vi "Lab Panel V4.85.vi"() -> ()   [LabVIEW 2013]
uses:
  <vilib>/Platform/TimedLoop/XDataNode/timing_clust.ctl
  <vilib>/Platform/TimedLoop/XDataNode/nitl_modes.ctl
  <vilib>/Platform/TimedLoop/XDataNode/wakeup.ctl
  Global display 1.vi
  Global 1.vi
  Global display 3.vi
  Global display 2.vi
  <vilib>/platform/TimedLoop/XDataNode/XDataNode.xnode
  <vilib>/Platform/TimedLoop/XDataNode/XDNodeRunTimeDep.lvlib
panel:
  out "TEMP":bool
  out "AI":bool
  in  "stop all":bool
  in  "ADMIN":bool
  in  "Tab Control 2":T1(tab)
  out "SIG LAB05-2":T2 {"PF" format="%.2f"; "AMPS" format="%.1f"}
  out "SIG LAB05-1":T2 {"PF" format="%.2f"; "AMPS" format="%.1f"}
  out "SIG LAB04-2":T2 {"PF" format="%.2f"; "AMPS" format="%.1f"}
  out "SIG LAB04-1":T2 {"PF" format="%.2f"; "AMPS" format="%.1f"}
  out "SIG LAB03-2":T2 {"PF" format="%.2f"; "AMPS" format="%.1f"}
  out "SIG LAB03-1":T2 {"PF" format="%.2f"; "AMPS" format="%.1f"}
  out "SIG LAB02-2":T2 {"PF" format="%.2f"; "AMPS" format="%.1f"}
  in  "RUN LAB01-1":bool
  in  "O/I  LAB05-1":bool
  in  "O/I  LAB05-2":bool
  in  "O/I  LAB04-1":bool
  in  "O/I  LAB04-2":bool
  in  "O/I  LAB02-1":bool
  in  "O/I  LAB02-2":bool
  in  "O/I  LAB01-2":bool
  in  "O/I  LAB01-1":bool
  in  "O/I  LAB03-1":bool
  in  "RUN LAB05-2":bool
  in  "RUN LAB05-1":bool
  in  "RUN LAB04-2":bool
  in  "RUN LAB04-1":bool
  in  "RUN LAB03-2":bool
  in  "RUN LAB03-1":bool
  in  "RUN LAB02-2":bool
  in  "RUN LAB02-1":bool
  in  "RUN LAB01-2":bool
  in  "SELECT LAB05-2":T3(radio)
  in  "SELECT LAB05-1":T3(radio)
  in  "SELECT LAB04-2":T3(radio)
  in  "SELECT LAB04-1":T3(radio)
  in  "SELECT LAB03-2":T3(radio)
  in  "SELECT LAB03-1":T3(radio)
  in  "SELECT LAB02-2":T3(radio)
  in  "SELECT LAB02-1":T3(radio)
  in  "SELECT LAB01-2":T3(radio)
  in  "SELECT LAB01-1":T3(radio)
  in  "O/I  LAB03-2":bool
  out "SIG LAB01-1":T2 {"PF" format="%.2f"; "AMPS" format="%.1f"}
  out "SIG LAB01-2":T2 {"PF" format="%.2f"; "AMPS" format="%.1f"}
  out "SIG LAB02-1":T2 {"PF" format="%.2f"; "AMPS" format="%.1f"}
  out "DISP LAB05-2":T4 {"MINS" format="%.2g"}
  out "DISP LAB05-1":T4 {"MINS" format="%.2g"}
  out "DISP LAB04-2":T4 {"MINS" format="%.2g"}
  out "DISP LAB04-1":T4 {"MINS" format="%.2g"}
  out "DISP LAB03-2":T4 {"MINS" format="%.2g"}
  out "DISP LAB03-1":T4 {"MINS" format="%.2g"}
  in  "SET LAB05-2":T5={"NAME"="", "DESCRIPTION"="", "CYCLES"=5.0, "T-RISE mins"=0.0, "T-RISE deg C"=0.0} {"CYCLES" min=5.0 step=1.0}
  in  "SET LAB05-1":T5={"NAME"="", "DESCRIPTION"="", "CYCLES"=5.0, "T-RISE mins"=0.0, "T-RISE deg C"=0.0} {"CYCLES" min=5.0 step=1.0}
  in  "SET LAB04-2":T5={"NAME"="", "DESCRIPTION"="", "CYCLES"=5.0, "T-RISE mins"=0.0, "T-RISE deg C"=0.0} {"CYCLES" min=5.0 step=1.0}
  in  "SET LAB04-1":T5={"NAME"="", "DESCRIPTION"="", "CYCLES"=5.0, "T-RISE mins"=0.0, "T-RISE deg C"=0.0} {"CYCLES" min=5.0 step=1.0}
  in  "SET LAB03-2":T5={"NAME"="", "DESCRIPTION"="", "CYCLES"=5.0, "T-RISE mins"=0.0, "T-RISE deg C"=0.0} {"CYCLES" min=5.0 step=1.0}
  in  "SET LAB03-1":T5={"NAME"="", "DESCRIPTION"="", "CYCLES"=5.0, "T-RISE mins"=0.0, "T-RISE deg C"=0.0} {"CYCLES" min=5.0 step=1.0}
  out "DISP LAB02-2":T4 {"MINS" format="%.2g"}
  out "DISP LAB02-1":T4 {"MINS" format="%.2g"}
  in  "SET LAB02-2":T5={"NAME"="", "DESCRIPTION"="", "CYCLES"=5.0, "T-RISE mins"=0.0, "T-RISE deg C"=0.0} {"CYCLES" min=5.0 step=1.0}
  in  "SET LAB02-1":T5={"NAME"="", "DESCRIPTION"="", "CYCLES"=5.0, "T-RISE mins"=0.0, "T-RISE deg C"=0.0} {"CYCLES" min=5.0 step=1.0}
  out "RESULT LAB05-2":bool
  out "RESULT LAB05-1":bool
  out "RESULT LAB04-2":bool
  out "RESULT LAB04-1":bool
  out "RESULT LAB03-2":bool
  out "RESULT LAB03-1":bool
  out "RESULT LAB02-2":bool
  out "RESULT LAB02-1":bool
  out "RESULT LAB01-2":bool
  out "RESULT LAB01-1":bool
  in  "SET LAB01-1":T5={"NAME"="", "DESCRIPTION"="", "CYCLES"=5.0, "T-RISE mins"=0.0, "T-RISE deg C"=0.0} {"CYCLES" min=5.0 step=1.0}
  in  "SET LAB01-2":T5={"NAME"="", "DESCRIPTION"="", "CYCLES"=5.0, "T-RISE mins"=0.0, "T-RISE deg C"=0.0} {"CYCLES" min=5.0 step=1.0}
  out "DISP LAB01-1":T4 {"MINS" format="%.2g"}
  out "DISP LAB01-2":T4 {"MINS" format="%.2f"}
  out "TEMP RISE LAB05-2":cluster{"TL":dbl, "TN":dbl}
  out "TEMP RISE LAB05-1":cluster{"TL":dbl, "TN":dbl}
  out "TEMP RISE LAB04-2":cluster{"TL":dbl, "TN":dbl}
  out "TEMP RISE LAB04-1":cluster{"TL":dbl, "TN":dbl}
  out "TEMP RISE LAB03-2":cluster{"TL":dbl, "TN":dbl}
  out "TEMP RISE LAB03-1":cluster{"TL":dbl, "TN":dbl}
  out "TEMP RISE LAB02-2":cluster{"TL":dbl, "TN":dbl}
  out "TEMP RISE LAB02-1":cluster{"TL":dbl, "TN":dbl}
  out "TEMP RISE LAB01-2":cluster{"TL":dbl, "TN":dbl}
  out "TEMP RISE LAB01-1":cluster{"TL":dbl, "TN":dbl}
  in  "JIG OFF TIME (S)":dbl=2.0 min=2.0 max=10.0 step=0.5 format="%.1g"
  in  "JIG ON TIME (S)":dbl=1.0 min=1.0 max=10.0 step=0.5 format="%.1g"
  out "JIG LAB05-2":bool
  out "JIG LAB05-1":bool
  out "JIG LAB04-2":bool
  out "JIG LAB04-1":bool
  out "JIG LAB03-2":bool
  out "JIG LAB03-1":bool
  out "JIG LAB02-2":bool
  out "JIG LAB02-1":bool
  out "JIG LAB01-2":bool
  out "JIG LAB01-1":bool
  out "TEMP START LAB01-1":cluster{"TL":dbl, "TN":dbl}
  out "TEMP START LAB02-1":cluster{"TL":dbl, "TN":dbl}
  out "TEMP START LAB03-1":cluster{"TL":dbl, "TN":dbl}
  out "TEMP START LAB04-1":cluster{"TL":dbl, "TN":dbl}
  out "TEMP START LAB01-2":cluster{"TL":dbl, "TN":dbl}
  out "TEMP START LAB02-2":cluster{"TL":dbl, "TN":dbl}
  out "TEMP START LAB03-2":cluster{"TL":dbl, "TN":dbl}
  out "TEMP START LAB04-2":cluster{"TL":dbl, "TN":dbl}
  out "TEMP START LAB05-2":cluster{"TL":dbl, "TN":dbl}
  out "TEMP START LAB05-1":cluster{"TL":dbl, "TN":dbl}
  out "LOG LAB05-2":string
  out "LOG LAB04-2":string
  out "LOG LAB03-2":string
  out "LOG LAB02-2":string
  out "LOG LAB01-2":string
  out "LOG LAB05-1":string
  out "LOG LAB04-1":string
  out "LOG LAB03-1":string
  out "LOG LAB02-1":string
  out "LOG LAB01-1":string
  out "TEST VOLTS CHART":dynamicdata(graph)
  in  "Select  Cycle":enum32{"ON CYCLE", "OFF CYCLE"}(radio)
  out "TEST AMPS CHART":dynamicdata(graph)
  out "TEMPERATURE (L) CHART":dynamicdata(graph)
  out "TEMPERATURE (N) CHART":dynamicdata(graph)
  out "Message":string
  in  "MAIL SETTINGS":T6
  out "MAIL REPORT":string
  in  "TO (string):":string
  in  "Send Mail Now":bool
  in  "Auto Mail Send":bool
  in  "Network Directory":path
  out "OFF LO5-1":dbl
  out "OFF LO5-1":dbl
  out "OFF LO4-2":dbl
  out "OFF LO4-1":dbl
  out "OFF LO3-2":dbl
  out "OFF LO3-1":dbl
  out "OFF LO2-1":dbl
  out "OFF LO2-1":dbl
  out "OFF LO1-2":dbl
  out "OFF LO1-1":dbl
  out "JIG RELAY CYCLES":T7
  out "ON L05-2":cluster{"amps":dbl, "volts":dbl, "pf":dbl}
  out "ON L05-1":cluster{"amps":dbl, "volts":dbl, "pf":dbl}
  out "FAIL LAB05-2":cluster{"LO":dbl, "HI":dbl}
  out "FAIL LAB05-1":cluster{"LO":dbl, "HI":dbl}
  out "FAIL LAB04-2":cluster{"LO":dbl, "HI":dbl}
  out "FAIL LAB04-1":cluster{"LO":dbl, "HI":dbl}
  out "FAIL LAB03-2":cluster{"LO":dbl, "HI":dbl}
  out "FAIL LAB03-1":cluster{"LO":dbl, "HI":dbl}
  out "FAIL LAB02-2":cluster{"LO":dbl, "HI":dbl}
  out "FAIL LAB02-1":cluster{"LO":dbl, "HI":dbl}
  out "FAIL LAB01-2":cluster{"LO":dbl, "HI":dbl}
  out "FAIL LAB01-1":cluster{"LO":dbl, "HI":dbl}
  out "ON L01-1":cluster{"amps":dbl, "volts":dbl, "pf":dbl}
  out "ON L01-2":cluster{"amps":dbl, "volts":dbl, "pf":dbl}
  out "ON L02-1":cluster{"amps":dbl, "volts":dbl, "pf":dbl}
  out "ON L02-2":cluster{"amps":dbl, "volts":dbl, "pf":dbl}
  out "ON L03-1":cluster{"amps":dbl, "volts":dbl, "pf":dbl}
  out "ON L03-2":cluster{"amps":dbl, "volts":dbl, "pf":dbl}
  out "ON L04-1":cluster{"amps":dbl, "volts":dbl, "pf":dbl}
  out "ON L04-2":cluster{"amps":dbl, "volts":dbl, "pf":dbl}
  out "TEMP LA05":T8
  out "TEMP LA04":T8
  out "TEMP LA03":T8
  out "TEMP LA02":T8
  out "TEMP LA01":T8
  in  "Test File To":string
  in  "Mail Test Fail":bool
  out "graph flag":bool
  in  "Temp Test Cal":dbl
  in  "spare":dbl
  out "Temp Loops":dbl
  in  "Fail Loops":dbl
  out "Save JC":bool
  out "simulate":bool
  in  "Temp Value":dbl
  in  "Temp Delay Lps":dbl
  in  "SAMPLES":dbl
  in  "RATE (Hz)":dbl
  in  "JIG TEST":T9
  in  "C drive data root dir":path
  out "run lab05-2":bool
  out "run lab05-1":bool
  out "run lab04-2":bool
  out "run lab04-1":bool
  out "run lab03-2":bool
  out "run lab03-1":bool
  out "run lab02-2":bool
  out "run lab02-1":bool
  out "run lab01-2":bool
  out "run lab01-1":bool
  in  "Tab Control":T10(tab)
  out "LAB01-2 (GRAPH)":dynamicdata(graph)
  out "LAB01-1 (GRAPH)":dynamicdata(graph)
  out "LAB02-2 (GRAPH)":dynamicdata(graph)
  out "LAB02-1 (GRAPH)":dynamicdata(graph)
  out "LAB03-2 (GRAPH)":dynamicdata(graph)
  out "LAB03-1 (GRAPH)":dynamicdata(graph)
  out "LAB04-2 (GRAPH)":dynamicdata(graph)
  out "LAB04-1 (GRAPH)":dynamicdata(graph)
  out "LAB05-2 (GRAPH)":dynamicdata(graph)
  out "LAB05-1 (GRAPH)":dynamicdata(graph)
  out "LAB05 TEMP":T11
  out "LAB04 TEMP":T11
  out "LAB02 TEMP":T11
  out "LAB01 TEMP":T11
  out "LAB03 TEMP":T11
  out "Analog Error Array":errorcluster[](array[cluster])
  out "AI loop time":dbl format="%.6g"
  out "loops":dbl
  in  "loop  delay(mS)":dbl
  out "on loops":dbl
  out "off loops":dbl
  out "jig cycle":dbl
  out "TDMS LAB01-1":refnum<k34>
  out "data file error":errorcluster
  out "TDMS LAB02-1":refnum<k34>
  out "TDMS LAB01-2":refnum<k34>
  out "TDMS LAB02-2":refnum<k34>
  out "TDMS LAB03-1":refnum<k34>
  out "TDMS LAB03-2":refnum<k34>
  out "TDMS LAB04-1":refnum<k34>
  out "TDMS LAB04-2":refnum<k34>
  out "TDMS LAB05-1":refnum<k34>
  out "TDMS LAB05-2":refnum<k34>
  out "mail control":string
  out "File Time Stamp":timestamp
  in  "stop":bool
  in  "Select COM port":refnum<visa-resource-name>="COM6"
  out "COM port":refnum<visa-resource-name>="COM6"
  out "CAL LAB01":T12 {"2 (TN) cal" min=0.0 step=0.01 format="%.2f"; "2 (TL) cal" min=0.0 step=0.01 format="%.2f"; "2 (PF) cal" min=0.0 step=0.01 format="%.2f"; "2 (V) cal" min=0.0 step=0.01 format="%.2f"; "2 (A) cal" min=0.0 step=0.01 format="%.2f"; "1 (TN) cal" min=0.0 step=0.01 format="%.2f"; "1 (TL) cal" min=0.0 step=0.01 format="%.2f"; "1 (PF) cal" min=0.0 step=0.01 format="%.2f"; "1 (V) cal" min=0.0 step=0.01 format="%.2f"; "1  (A) cal" min=0.0 step=0.01 format="%.2f"}
  out "CAL LAB03":T12 {"2 (TN) cal" min=0.0 step=0.01 format="%.2f"; "2 (TL) cal" min=0.0 step=0.01 format="%.2f"; "2 (PF) cal" min=0.0 step=0.01 format="%.2f"; "2 (V) cal" min=0.0 step=0.01 format="%.2f"; "2 (A) cal" min=0.0 step=0.01 format="%.2f"; "1 (TN) cal" min=0.0 step=0.01 format="%.2f"; "1 (TL) cal" min=0.0 step=0.01 format="%.2f"; "1 (PF) cal" min=0.0 step=0.01 format="%.2f"; "1 (V) cal" min=0.0 step=0.01 format="%.2f"; "1  (A) cal" min=0.0 step=0.01 format="%.2f"}
  out "CAL LAB02":T13 {"2 (TN) cal" min=0.0 step=0.01 format="%.2f"; "2 (TL) cal" min=0.0 step=0.01 format="%.2f"; "2 (PF) cal" min=0.0 step=0.01 format="%.2f"; "2 (V) cal" min=0.0 step=0.01 format="%.2f"; "2 (A) cal" min=0.0 step=0.01 format="%.2f"; "1 (TN) cal" min=0.0 step=0.01 format="%.2f"; "1 (TL) cal" min=0.0 step=0.01 format="%.2f"; "1 (PF) cal" min=0.0 step=0.01 format="%.2f"; "1 (V) cal" min=0.0 step=0.01 format="%.2f"; "1 (A) cal" min=0.0 step=0.01 format="%.2f"}
  out "CAL LAB05":T12 {"2 (TN) cal" min=0.0 step=0.01 format="%.2f"; "2 (TL) cal" min=0.0 step=0.01 format="%.2f"; "2 (PF) cal" min=0.0 step=0.01 format="%.2f"; "2 (V) cal" min=0.0 step=0.01 format="%.2f"; "2 (A) cal" min=0.0 step=0.01 format="%.2f"; "1 (TN) cal" min=0.0 step=0.01 format="%.2f"; "1 (TL) cal" min=0.0 step=0.01 format="%.2f"; "1 (PF) cal" min=0.0 step=0.01 format="%.2f"; "1 (V) cal" min=0.0 step=0.01 format="%.2f"; "1  (A) cal" min=0.0 step=0.01 format="%.2f"}
  out "CAL LAB04":T12 {"2 (TN) cal" min=0.0 step=0.01 format="%.2f"; "2 (TL) cal" min=0.0 step=0.01 format="%.2f"; "2 (PF) cal" min=0.0 step=0.01 format="%.2f"; "2 (V) cal" min=0.0 step=0.01 format="%.2f"; "2 (A) cal" min=0.0 step=0.01 format="%.2f"; "1 (TN) cal" min=0.0 step=0.01 format="%.2f"; "1 (TL) cal" min=0.0 step=0.01 format="%.2f"; "1 (PF) cal" min=0.0 step=0.01 format="%.2f"; "1 (V) cal" min=0.0 step=0.01 format="%.2f"; "1  (A) cal" min=0.0 step=0.01 format="%.2f"}
  out "cal file error out":errorcluster
  in  "SET (cal)":bool
  # "LAB01"
  # "LAB02"
  # "LAB03"
  # "LAB04"
  # "LAB05"
  # "LAB01"
  # "LAB02"
  # "LAB03"
  # "LAB04"
  # "LAB05"
  # "JIG SET"
  # "PANEL ID / DATE / TIME / DESCRIPTION / CYCLES / TEST TIME / STATUS"
  # "PANEL ID / DATE / TIME / DESCRIPTION / CYCLES / TEST TIME / STATUS"
  # "(Enter recipients address seperated by comma)"
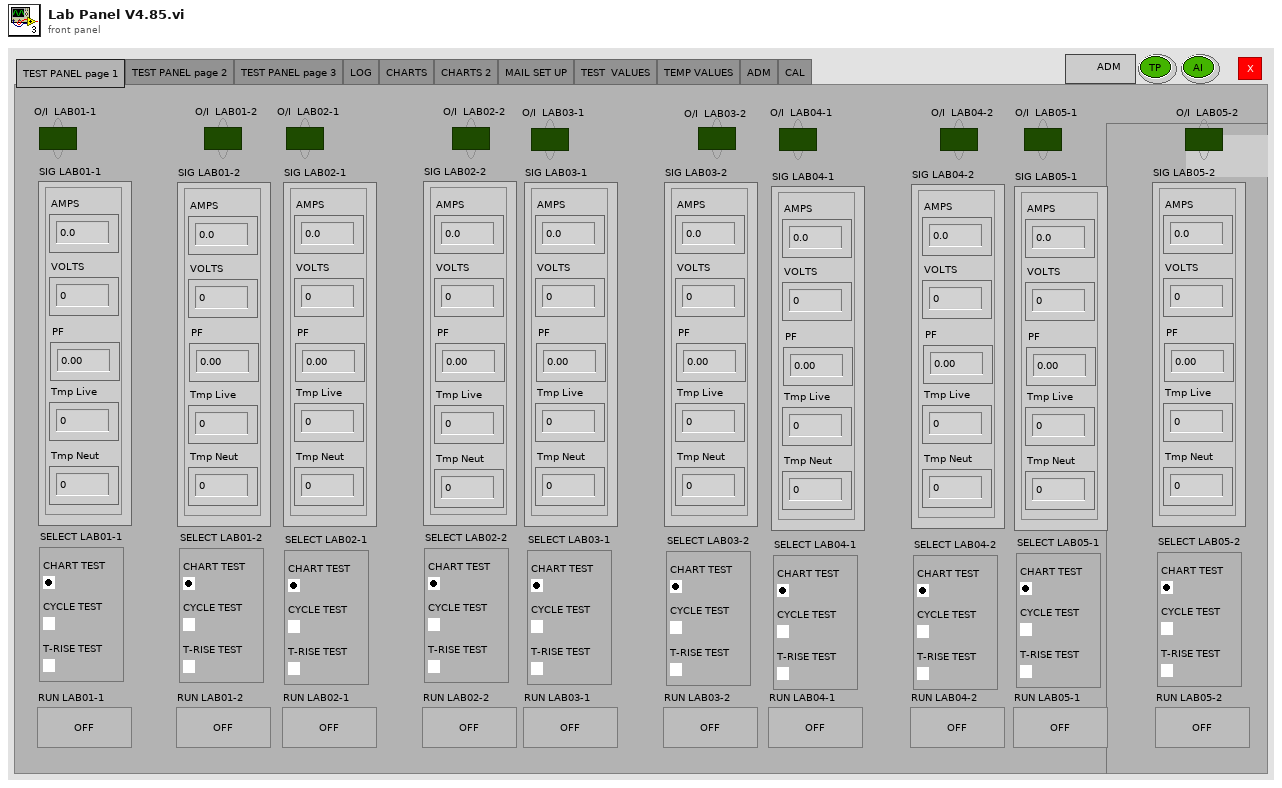
[diagram p1: front panel]
types:
  T1 = enum32{"TEST PANEL page 1", "TEST PANEL page 2", "TEST PANEL page 3", "LOG", "CHARTS", "CHARTS 2", "MAIL SET UP", "TEST  VALUES", "TEMP VALUES", "ADM", "CAL"}
  T2 = cluster{"AMPS":dbl, "VOLTS":dbl, "PF":dbl, "Tmp Live":dbl, "Tmp Neut":dbl}
  T3 = enum32{"CHART TEST", "CYCLE TEST", "T-RISE TEST"}
  T4 = cluster{"CYCLE":dbl, "MINS":dbl, "STATUS":string}
  T5 = cluster{"NAME":string, "DESCRIPTION":string, "CYCLES":dbl, "T-RISE mins":dbl, "T-RISE deg C":dbl}
  T6 = cluster{"OUT SERVER ADDRESS":string, "FROM ACCOUNT":string, "USER NAME":string, "PASSWORD":string, "TEST MAIL":bool, "TEST MAIL STATUS":string, "mail error":errorcluster}
  T7 = cluster{"LAB01-1":dbl, "LAB01-2":dbl, "LAB02-1":dbl, "LAB02-2":dbl, "LAB03-1":dbl, "LAB03-2":dbl, "LAB04-1":dbl, "LAB04-2":dbl, "LAB05-1":dbl, "LAB05-2":dbl}
  T8 = cluster{"TL-1":dbl, "TN-1":dbl, "TL-2":dbl, "TN-2":dbl, "TL -1COUNT":dbl, "TN-1 COUNT":dbl, "TL-2 COUNT":dbl, "TN-2 COUNT":dbl}
  T9 = cluster{" LAB01-1":bool, " LAB01-2":bool, "LAB02-1":bool, " LAB02-2":bool, "LAB03-1":bool, "LAB03-2":bool, "LAB04-1":bool, "LAB04-2":bool, "LAB05-1":bool, "LAB05-2":bool}
  T10 = enum32{"LAB01", "LAB02", "LAB03", "LAB04", "LAB05", "TEMPERATURE", "ERROR"}
  T11 = cluster{"T1 Live":dbl, "T1 Neut":dbl, "T2 Live":dbl, "T2 Neut":dbl, "ID":dbl, "ER":dbl}
  T12 = cluster{"1  (A) cal":dbl, "1 (V) cal":dbl, "1 (PF) cal":dbl, "1 (TL) cal":dbl, "1 (TN) cal":dbl, "2 (A) cal":dbl, "2 (V) cal":dbl, "2 (PF) cal":dbl, "2 (TL) cal":dbl, "2 (TN) cal":dbl}
  T13 = cluster{"1 (A) cal":dbl, "1 (V) cal":dbl, "1 (PF) cal":dbl, "1 (TL) cal":dbl, "1 (TN) cal":dbl, "2 (A) cal":dbl, "2 (V) cal":dbl, "2 (PF) cal":dbl, "2 (TL) cal":dbl, "2 (TN) cal":dbl}
  T14 = enum8{"Enabled", "Disabled", "Disabled and Grayed Out"}
  T15 = typedef "XDNodeRunTimeDep.lvlib/timing_clust.ctl" = cluster{"Expected End [f-1]":u64, "Actual End [f-1]":u64, "Finished Late? [f-1]":bool, "Expected End [i-1]":u64, "Actual End [i-1]":u64, "Finished Late? [i-1]":bool, "Expected Start [i]":u64, "Actual Start [i]":u64, "Expected Start [f]":u64, "Actual Start [f]":u64, "Source Name":string, "Structure Name":string, "Period":i64, "Deadline":i64, "Offset":i64, "Start":i64, "Priority":i32, "Timeout":i32, "Mode":T16, "Wakeup Reason":T17, "Error":errorcluster, "Source Type":string, "Secondary Source Type":string, "Global End Time":u64, "Global Start Time":u64, "Frame Duration":u64, "Iteration Duration":u64, "Assigned CPU":i32, "I/O Scan Engine Mode":u32}
  T16 = typedef "XDNodeRunTimeDep.lvlib/nitl_modes.ctl" = enum32{"No Change", "Process missed periods, maintain original phase", "Discard missed periods, maintain original phase", "Process missed periods, ignore original phase", "Discard missed periods, ignore original phase"}
  T17 = typedef "XDNodeRunTimeDep.lvlib/wakeup.ctl" = enum32{"Normal", "Aborted", "Asynchronous wakeup", "Timing source error", "Timed loop error", "Timeout"}
  T18 = enum16{"open", "open or create", "create or replace", "create", "open (read-only)"}
  T19 = enum16{"open", "replace", "create", "open or create", "replace or create", "replace or create with confirmation"}
  T20 = cluster{"SET LAB01-1":cluster{"NAME":string, "DESCRIPTION":string, "CYCLES":dbl, "T-RISE mins":dbl, "T-RISE deg C":dbl}, "SET LAB01-2":cluster{"NAME":string, "DESCRIPTION":string, "CYCLES":dbl, "T-RISE mins":dbl, "T-RISE deg C":dbl}, "SET LAB02-1":cluster{"NAME":string, "DESCRIPTION":string, "CYCLES":dbl, "T-RISE mins":dbl, "T-RISE deg C":dbl}, "SET LAB02-2":cluster{"NAME":string, "DESCRIPTION":string, "CYCLES":dbl, "T-RISE mins":dbl, "T-RISE deg C":dbl}, "SET LAB03-1":cluster{"NAME":string, "DESCRIPTION":string, "CYCLES":dbl, "T-RISE mins":dbl, "T-RISE deg C":dbl}, "SET LAB03-2":cluster{"NAME":string, "DESCRIPTION":string, "CYCLES":dbl, "T-RISE mins":dbl, "T-RISE deg C":dbl}, "SET LAB04-1":cluster{"NAME":string, "DESCRIPTION":string, "CYCLES":dbl, "T-RISE mins":dbl, "T-RISE deg C":dbl}, "SET LAB04-2":cluster{"NAME":string, "DESCRIPTION":string, "CYCLES":dbl, "T-RISE mins":dbl, "T-RISE deg C":dbl}, "SET LAB05-1":cluster{"NAME":string, "DESCRIPTION":string, "CYCLES":dbl, "T-RISE mins":dbl, "T-RISE deg C":dbl}, "SET LAB05-2":cluster{"NAME":string, "DESCRIPTION":string, "CYCLES":dbl, "T-RISE mins":dbl, "T-RISE deg C":dbl}, "Network Directory":path, "C drive data root dir":path, "RATE (Hz)":dbl, "SAMPLES":dbl, "Select COM port":refnum<visa-resource-name>, "Temp Delay Lps":dbl, "Temp Value":dbl, "Fail Loops":dbl, "Temp Test Cal":dbl, "spare":dbl, "Test File To":string, "Mail Test Fail":bool}
  T21 = cluster{"MAIL SETTINGS":cluster{"OUT SERVER ADDRESS":string, "FROM ACCOUNT":string, "USER NAME":string, "PASSWORD":string, "TEST MAIL":bool, "TEST MAIL STATUS":string, "mail error":errorcluster}, "Auto Mail Send":bool, string}
  T22 = cluster{"T1":dbl, "T2":dbl, "T3":dbl, "T4":dbl, "ID":dbl, "ER":dbl}
  T23 = cluster{"STATUS":string, "OUT SERVER ADDRESS":string, "FROM ACCOUNT":string, "Test File To":string, "Mail Test Fail":bool}
  T24 = cluster{"LAB01-1 (A)":dbl, "LAB01-1 (V)":dbl, "LAB01-1 (PF)":dbl, "LAB01-2 (A)":dbl, "LAB01-2 (V)":dbl, "LAB01-2 (PF)":dbl}
  T25 = cluster{"LAB02-1 (A)":dbl, "LAB02-1 (V)":dbl, "LAB02-1 (PF)":dbl, "LAB02-2 (A)":dbl, "LAB02-2 (V)":dbl, "LAB02-2 (PF)":dbl}
  T26 = cluster{"LAB03-1 (A)":dbl, "LAB03-1 (V)":dbl, "LAB03-1 (PF)":dbl, "LAB03-2 (A)":dbl, "LAB03-2 (V)":dbl, "LAB03-2 (PF)":dbl}
  T27 = cluster{"LAB04-1 (A)":dbl, "LAB04-1 (V)":dbl, "LAB04-1 (PF)":dbl, "LAB04-2 (A)":dbl, "LAB04-2 (V)":dbl, "LAB04-2 (PF)":dbl}
  T28 = cluster{"LAB05-1 (A)":dbl, "LAB05-1 (V)":dbl, "LAB05-1 (PF)":dbl, "LAB05-2 (A)":dbl, "LAB05-2 (V)":dbl, "LAB05-2 (PF)":dbl}
  T29 = cluster{"FAIL LAB01-1":cluster{"LO":dbl, "HI":dbl}, "SIG LAB01-1":cluster{"AMPS":dbl, "VOLTS":dbl, "PF":dbl, "Tmp Live":dbl, "Tmp Neut":dbl}, "TEMP START LAB01-1":cluster{"TL":dbl, "TN":dbl}, "DISP LAB01-1":cluster{"CYCLE":dbl, "MINS":dbl, "STATUS":string}, "SET LAB01-1":cluster{"NAME":string, "DESCRIPTION":string, "CYCLES":dbl, "T-RISE mins":dbl, "T-RISE deg C":dbl}, "TDMS LAB01-1":refnum<k34>}
  T30 = cluster{"FAIL LAB01-2":cluster{"LO":dbl, "HI":dbl}, "SIG LAB01-2":cluster{"AMPS":dbl, "VOLTS":dbl, "PF":dbl, "Tmp Live":dbl, "Tmp Neut":dbl}, "TEMP START LAB01-2":cluster{"TL":dbl, "TN":dbl}, "DISP LAB01-2":cluster{"CYCLE":dbl, "MINS":dbl, "STATUS":string}, "SET LAB01-2":cluster{"NAME":string, "DESCRIPTION":string, "CYCLES":dbl, "T-RISE mins":dbl, "T-RISE deg C":dbl}, "TDMS LAB01-2":refnum<k34>}
  T31 = cluster{"FAIL LAB02-1":cluster{"LO":dbl, "HI":dbl}, "SIG LAB02-1":cluster{"AMPS":dbl, "VOLTS":dbl, "PF":dbl, "Tmp Live":dbl, "Tmp Neut":dbl}, "TEMP START LAB02-1":cluster{"TL":dbl, "TN":dbl}, "DISP LAB02-1":cluster{"CYCLE":dbl, "MINS":dbl, "STATUS":string}, "SET LAB02-1":cluster{"NAME":string, "DESCRIPTION":string, "CYCLES":dbl, "T-RISE mins":dbl, "T-RISE deg C":dbl}, "TDMS LAB02-1":refnum<k34>}
  T32 = cluster{"FAIL LAB02-2":cluster{"LO":dbl, "HI":dbl}, "SIG LAB02-2":cluster{"AMPS":dbl, "VOLTS":dbl, "PF":dbl, "Tmp Live":dbl, "Tmp Neut":dbl}, "TEMP START LAB02-2":cluster{"TL":dbl, "TN":dbl}, "DISP LAB02-2":cluster{"CYCLE":dbl, "MINS":dbl, "STATUS":string}, "SET LAB02-2":cluster{"NAME":string, "DESCRIPTION":string, "CYCLES":dbl, "T-RISE mins":dbl, "T-RISE deg C":dbl}, "TDMS LAB02-2":refnum<k34>}
  T33 = cluster{"FAIL LAB03-1":cluster{"LO":dbl, "HI":dbl}, "SIG LAB03-1":cluster{"AMPS":dbl, "VOLTS":dbl, "PF":dbl, "Tmp Live":dbl, "Tmp Neut":dbl}, "TEMP START LAB03-1":cluster{"TL":dbl, "TN":dbl}, "DISP LAB03-1":cluster{"CYCLE":dbl, "MINS":dbl, "STATUS":string}, "SET LAB03-1":cluster{"NAME":string, "DESCRIPTION":string, "CYCLES":dbl, "T-RISE mins":dbl, "T-RISE deg C":dbl}, "TDMS LAB03-1":refnum<k34>}
  T34 = cluster{"FAIL LAB03-2":cluster{"LO":dbl, "HI":dbl}, "SIG LAB03-2":cluster{"AMPS":dbl, "VOLTS":dbl, "PF":dbl, "Tmp Live":dbl, "Tmp Neut":dbl}, "TEMP START LAB03-2":cluster{"TL":dbl, "TN":dbl}, "DISP LAB03-2":cluster{"CYCLE":dbl, "MINS":dbl, "STATUS":string}, "SET LAB03-2":cluster{"NAME":string, "DESCRIPTION":string, "CYCLES":dbl, "T-RISE mins":dbl, "T-RISE deg C":dbl}, "TDMS LAB03-2":refnum<k34>}
  T35 = cluster{"FAIL LAB04-1":cluster{"LO":dbl, "HI":dbl}, "SIG LAB04-1":cluster{"AMPS":dbl, "VOLTS":dbl, "PF":dbl, "Tmp Live":dbl, "Tmp Neut":dbl}, "TEMP START LAB04-1":cluster{"TL":dbl, "TN":dbl}, "DISP LAB04-1":cluster{"CYCLE":dbl, "MINS":dbl, "STATUS":string}, "SET LAB04-1":cluster{"NAME":string, "DESCRIPTION":string, "CYCLES":dbl, "T-RISE mins":dbl, "T-RISE deg C":dbl}, "TDMS LAB04-1":refnum<k34>}
  T36 = cluster{"FAIL LAB04-2":cluster{"LO":dbl, "HI":dbl}, "SIG LAB04-2":cluster{"AMPS":dbl, "VOLTS":dbl, "PF":dbl, "Tmp Live":dbl, "Tmp Neut":dbl}, "TEMP START LAB04-2":cluster{"TL":dbl, "TN":dbl}, "DISP LAB04-2":cluster{"CYCLE":dbl, "MINS":dbl, "STATUS":string}, "SET LAB04-2":cluster{"NAME":string, "DESCRIPTION":string, "CYCLES":dbl, "T-RISE mins":dbl, "T-RISE deg C":dbl}, "TDMS LAB04-2":refnum<k34>}
  T37 = cluster{"FAIL LAB05-1":cluster{"LO":dbl, "HI":dbl}, "SIG LAB05-1":cluster{"AMPS":dbl, "VOLTS":dbl, "PF":dbl, "Tmp Live":dbl, "Tmp Neut":dbl}, "TEMP START LAB05-1":cluster{"TL":dbl, "TN":dbl}, "DISP LAB05-1":cluster{"CYCLE":dbl, "MINS":dbl, "STATUS":string}, "SET LAB05-1":cluster{"NAME":string, "DESCRIPTION":string, "CYCLES":dbl, "T-RISE mins":dbl, "T-RISE deg C":dbl}, "TDMS LAB05-1":refnum<k34>}
  T38 = cluster{"FAIL LAB05-2":cluster{"LO":dbl, "HI":dbl}, "SIG LAB05-2":cluster{"AMPS":dbl, "VOLTS":dbl, "PF":dbl, "Tmp Live":dbl, "Tmp Neut":dbl}, "TEMP START LAB05-2":cluster{"TL":dbl, "TN":dbl}, "DISP LAB05-2":cluster{"CYCLE":dbl, "MINS":dbl, "STATUS":string}, "SET LAB05-2":cluster{"NAME":string, "DESCRIPTION":string, "CYCLES":dbl, "T-RISE mins":dbl, "T-RISE deg C":dbl}, "TDMS LAB05-2":refnum<k34>}
  T39 = cluster{"MAIL SETTINGS":cluster{"OUT SERVER ADDRESS":string, "FROM ACCOUNT":string, "USER NAME":string, "PASSWORD":string, "TEST MAIL":bool, "TEST MAIL STATUS":string, "mail error":errorcluster}, "Auto Mail Send":bool, "TO (string):":string}
  T40 = cluster{"TP1-L":dbl, "TP1-N":dbl, "TP2-L":dbl, "TP2-N":dbl, "TP1-L COUNT":dbl, "TP1-N COUNT":dbl, "TP2-L COUNT":dbl, "TP2-N COUNT":dbl}
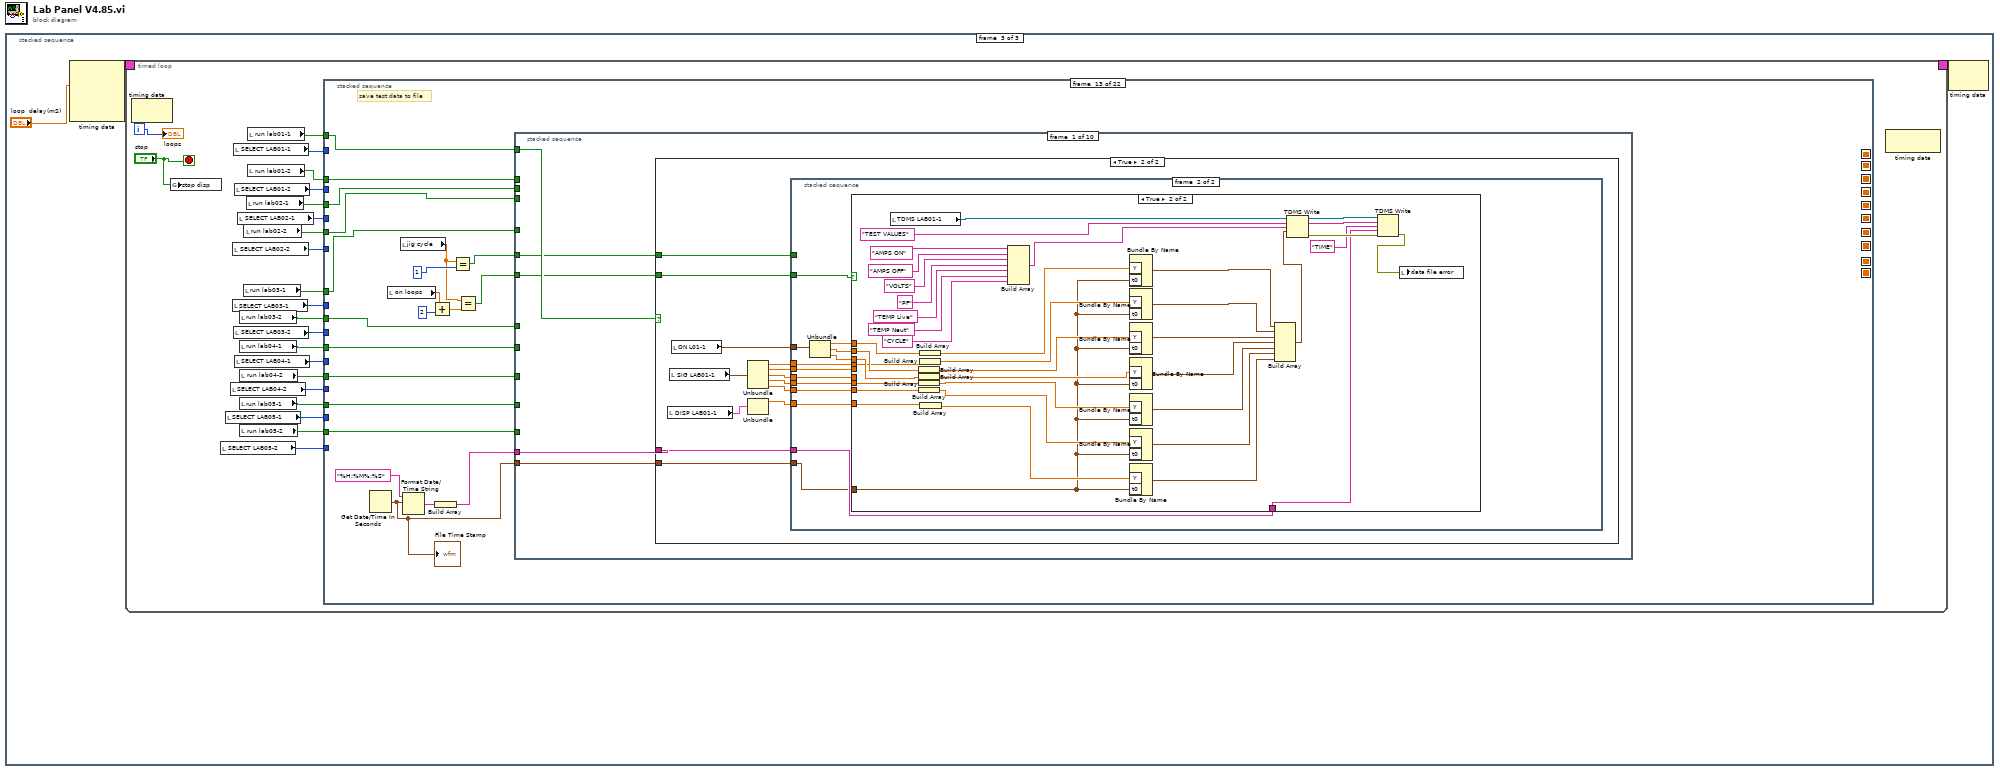
[diagram p0: block diagram]
diagram:
  n1 = stacked-sequence {
    frame #0 {
      n2 = local write "loop  delay(mS)"(500) -> ()
      n3 = local write "Save JC"(FALSE) -> ()
      "jig cycle" <- 0
    }
    frame #1 {
      # "do 1st time set up"
      n4 = stacked-sequence {
        frame #0 {
          # "disable front panel while 1st time set up is being done"
          n5 = disable-structure shown="Enabled" {
            frame Enabled {
              n6 = property on="Tab Control 2" class="TabCtl (strict)"() -> ("Pages"=w10:refnum<vi>[])  [unwired: 2 in, 2 out]
              n7 = Index Array(array=w10, index=9) -> (element=w8:refnum<vi>)
              n8 = property class="Page"(reference=w8, "PageVis"=FALSE) -> ()  [unwired: 1 in, 2 out]
            }
            frame Disabled {
            }
          }
          n9 = property on="Tab Control 2" class="TabCtl (strict)"("Value"=0) -> ()  [unwired: 2 in, 2 out]
          n10 = local write "ADMIN"(FALSE) -> ()
          n11 = property on="Tab Control 2" class="TabCtl (strict)"("DisabledEnum"=T14."Disabled and Grayed Out" ("Disabled")) -> ()  [unwired: 2 in, 2 out]
        }
        frame #1 {
          # "get calibration values"
          n12 = call "sub vi - get calibration values v1.vi"() -> ("LAB01 (CAL)"=→"CAL LAB01":T12, "LAB02 (CAL)"=→"CAL LAB02":T13, "LAB03 (CAL)"=→"CAL LAB03":T12, "LAB04 (CAL)"=→"CAL LAB04":T12, "calibration file error out"=→"cal file error out":errorcluster, "LAB05 (CAL)"=→"CAL LAB05":T12)  [unwired: 10 in]
        }
        frame #2 {
          # "get last saved test settings from file"
          n13 = local read "Network Directory"() -> (w39:path)
          n14 = local read "C drive data root dir"() -> (w37:path)
          n15 = local read "SET LAB05-2"() -> (w69:T5)
          n16 = local read "SET LAB05-1"() -> (w70:T5)
          n17 = local read "SAMPLES"() -> (w35:dbl)
          n18 = local read "SET LAB04-2"() -> (w71:T5)
          n19 = local read "RATE (Hz)"() -> (w36:dbl)
          n20 = local read "SET LAB03-2"() -> (w68:T5)
          n21 = local read "SET LAB04-1"() -> (w72:T5)
          n22 = local read "SET LAB03-1"() -> (w67:T5)
          n23 = local read "SET LAB02-2"() -> (w66:T5)
          n24 = local read "SET LAB02-1"() -> (w65:T5)
          n25 = local read "SET LAB01-2"() -> (w64:T5)
          n26 = local read "SET LAB01-1"() -> (w63:T5)
          n27 = local read "Select COM port"() -> (w31:refnum<visa-resource-name>)
          n28 = local read "Temp Delay Lps"() -> (w30:dbl)
          n29 = local read "Temp Value"() -> (w29:dbl)
          n30 = local read "Temp Test Cal"() -> (w24:dbl)
          n31 = local read "Test File To"() -> (w20:string)
          n32 = local read "Fail Loops"() -> (w26:dbl)
          n33 = local read "Mail Test Fail"() -> (w18:bool)
          n34 = local read "spare"() -> (w23:dbl)
          n35 = Bundle("SET LAB01-1"=w63, "SET LAB01-2"=w64, "SET LAB02-1"=w65, "SET LAB02-2"=w66, "SET LAB03-1"=w67, "SET LAB03-2"=w68, "SET LAB04-1"=w72, "SET LAB04-2"=w71, "SET LAB05-1"=w70, "SET LAB05-2"=w69, "Network Directory"=w39, "C drive data root dir"=w37, "RATE (Hz)"=w36, "SAMPLES"=w35, "Select COM port"=w31, "Temp Delay Lps"=w30, "Temp Value"=w29, "Fail Loops"=w26, "Temp Test Cal"=w24, "spare"=w23, "Test File To"=w20, "Mail Test Fail"=w18) -> (w56:T20)  [unwired: 1 in]
          n36 = String To Path(string="c:\\crabtree\\Set Up\\") -> (path=w60:path)
          n37 = Build Path(base path=w60, name or relative path="settings.bin") -> (appended path=w58:path)
          n38 = Create Folder(path (use dialog)=w60) -> (error out=w62:errorcluster)  [unwired: 2 in, 2 out]
          n39 = call <vilib>:"Clear Errors.vi"("error in (no error)"=w62) -> ()  [unwired: 6 in, 1 out]
          n40 = Open/Create/Replace File(file path (use dialog)=w58) -> (refnum out=w55:refnum<file>, error out=w57:errorcluster)  [unwired: 5 in, 1 out]
          n41 = Read from Binary File(5:w56, 8:w57, 11:w55) -> (0:w52:errorcluster, 2:w54:T20, 3:w53:refnum<file>)  [unwired: 3 in, 1 out]
          n42 = Unbundle(w54) -> ("SET LAB01-1"=w50:T5, "SET LAB01-2"=w49:T5, "SET LAB02-1"=w48:T5, "SET LAB02-2"=w47:T5, "SET LAB03-1"=w46:T5, "SET LAB03-2"=w45:T5, "SET LAB04-1"=w44:T5, "SET LAB04-2"=w43:T5, "SET LAB05-1"=w42:T5, "SET LAB05-2"=w41:T5, "Network Directory"=w40:path, "C drive data root dir"=w38:path, "RATE (Hz)"=w33:dbl, "SAMPLES"=w34:dbl, "Select COM port"=w32:refnum<visa-resource-name>, "Temp Delay Lps"=w28:dbl, "Temp Value"=w27:dbl, "Fail Loops"=w25:dbl, "Temp Test Cal"=w22:dbl, "spare"=w21:dbl, "Test File To"=w19:string, "Mail Test Fail"=w17:bool)
          n43 = Close File(refnum=w53, error in=w52) -> (error out=w51:errorcluster)  [unwired: 1 out]
          n44 = local write "data file error"(w51) -> ()
          n45 = local write "Temp Test Cal"(w22) -> ()
          n46 = local write "Mail Test Fail"(w17) -> ()
          n47 = local write "Test File To"(w19) -> ()
          n48 = local write "Fail Loops"(w25) -> ()
          n49 = local write "Temp Delay Lps"(w28) -> ()
          n50 = local write "C drive data root dir"(w38) -> ()
          n51 = local write "spare"(w21) -> ()
          n52 = local write "Temp Value"(w27) -> ()
          n53 = local write "Select COM port"(w32) -> ()
          n54 = local write "Network Directory"(w40) -> ()
          n55 = local write "SAMPLES"(w34) -> ()
          n56 = local write "RATE (Hz)"(w33) -> ()
          n57 = local write "SET LAB04-2"(w43) -> ()
          n58 = local write "SET LAB05-1"(w42) -> ()
          n59 = local write "SET LAB04-1"(w44) -> ()
          n60 = local write "SET LAB05-2"(w41) -> ()
          n61 = local write "SET LAB02-1"(w48) -> ()
          n62 = local write "SET LAB02-2"(w47) -> ()
          n63 = local write "SET LAB03-1"(w46) -> ()
          n64 = local write "SET LAB03-2"(w45) -> ()
          n65 = local write "SET LAB01-1"(w50) -> ()
          n66 = local write "SET LAB01-2"(w49) -> ()
        }
        frame #3 {
          # "get last saved jig cycles value from file"
          n67 = String To Path(string="c:\\crabtree\\Jig Cycles\\") -> (path=w82:path)
          n68 = Build Path(base path=w82, name or relative path="jigcycles.bin") -> (appended path=w80:path)
          n69 = Create Folder(path (use dialog)=w82) -> (error out=w84:errorcluster)  [unwired: 2 in, 2 out]
          n70 = call <vilib>:"Clear Errors.vi"("error in (no error)"=w84) -> ()  [unwired: 6 in, 1 out]
          n71 = Open/Create/Replace File(file path (use dialog)=w80) -> (refnum out=w78:refnum<file>, error out=w79:errorcluster)  [unwired: 5 in, 1 out]
          n72 = Read from Binary File(5:T7 {"LAB01-1"=0.0, "LAB01-2"=0.0, "LAB02-1"=0.0, "LAB02-2"=0.0, "LAB03-1"=0.0, "LAB03-2"=0.0, "LAB04-1"=0.0, "LAB04-2"=0.0, "LAB05-1"=0.0, "LAB05-2"=0.0} ("JIG RELAY CYCLES"), 8:w79, 11:w78) -> (0:w76:errorcluster, 2:w73:T7, 3:w77:refnum<file>)  [unwired: 3 in, 1 out]
          n73 = local write "JIG RELAY CYCLES"(w73) -> ()
          n74 = Close File(refnum=w77, error in=w76) -> (error out=w75:errorcluster)  [unwired: 1 out]
          n75 = local write "data file error"(w75) -> ()
        }
        frame #4 {
          # "get mail settings"
          n76 = local read "Auto Mail Send"() -> (w88:bool)
          n77 = local read "MAIL SETTINGS"() -> (w92:T6)
          n78 = String To Path(string="c:\\crabtree\\Set Up\\") -> (path=w100:path)
          n79 = Build Path(base path=w100, name or relative path="mail.bin") -> (appended path=w98:path)
          n80 = Create Folder(path (use dialog)=w100) -> (error out=w102:errorcluster)  [unwired: 2 in, 2 out]
          n81 = Bundle("MAIL SETTINGS"=w92, "Auto Mail Send"=w88, "") -> (w91:T21)  [unwired: 1 in]
          n82 = call <vilib>:"Clear Errors.vi"("error in (no error)"=w102) -> ()  [unwired: 6 in, 1 out]
          n83 = Open/Create/Replace File(file path (use dialog)=w98) -> (refnum out=w96:refnum<file>, error out=w97:errorcluster)  [unwired: 5 in, 1 out]
          n84 = Read from Binary File(5:w91, 8:w97, 11:w96) -> (0:w94:errorcluster, 2:w90:T21, 3:w95:refnum<file>)  [unwired: 3 in, 1 out]
          n85 = Unbundle(w90) -> ("MAIL SETTINGS"=w89:T6, "Auto Mail Send"=w87:bool, w86:string)
          n86 = local write "TO (string):"(w86) -> ()
          n87 = local write "Auto Mail Send"(w87) -> ()
          n88 = local write "MAIL SETTINGS"(w89) -> ()
          n89 = Close File(refnum=w95, error in=w94) -> (error out=w93:errorcluster)  [unwired: 1 out]
          n90 = local write "data file error"(w93) -> ()
        }
        frame #5 {
          # "set display status if blank"
          n91 = local read "DISP LAB03-2"() -> (w132:T4)
          n92 = local read "DISP LAB03-1"() -> (w139:T4)
          n93 = local read "DISP LAB02-2"() -> (w146:T4)
          n94 = local read "DISP LAB01-2"() -> (w159:T4)
          n95 = local read "DISP LAB01-1"() -> (w168:T4)
          n96 = local read "DISP LAB02-1"() -> (w153:T4)
          n97 = Unbundle(w132) -> ("STATUS"=w134:string)  [unwired: 2 out]
          n98 = Unbundle(w139) -> ("STATUS"=w141:string)  [unwired: 2 out]
          n99 = Unbundle(w146) -> ("STATUS"=w148:string)  [unwired: 2 out]
          n100 = Unbundle(w153) -> ("STATUS"=w155:string)  [unwired: 2 out]
          n101 = Unbundle(w159) -> ("STATUS"=w162:string)  [unwired: 2 out]
          n102 = Unbundle(w168) -> ("STATUS"=w169:string)  [unwired: 2 out]
          n103 = Equal?(x="", y=w134) -> (x = y?=w136:bool)
          n104 = Equal?(x="", y=w141) -> (x = y?=w143:bool)
          n105 = Equal?(x="", y=w148) -> (x = y?=w150:bool)
          n106 = Equal?(x="", y=w155) -> (x = y?=w157:bool)
          n107 = Equal?(x="", y=w162) -> (x = y?=w164:bool)
          n108 = Equal?(x="", y=w169) -> (x = y?=w171:bool)
          n109 = Select(t="STOP", s=w136, f=w134) -> (s? t:f=w133:string)
          n110 = Select(t="STOP", s=w143, f=w141) -> (s? t:f=w140:string)
          n111 = Select(t="STOP", s=w150, f=w148) -> (s? t:f=w147:string)
          n112 = Select(t="STOP", s=w157, f=w155) -> (s? t:f=w154:string)
          n113 = Select(t="STOP", s=w164, f=w162) -> (s? t:f=w161:string)
          n114 = Select(t="STOP", s=w171, f=w169) -> (s? t:f=w167:string)
          n115 = Bundle(cluster=w132, "STATUS"=w133) -> (w131:T4)  [unwired: 2 in]
          n116 = Bundle(cluster=w139, "STATUS"=w140) -> (w138:T4)  [unwired: 2 in]
          n117 = Bundle(cluster=w146, "STATUS"=w147) -> (w145:T4)  [unwired: 2 in]
          n118 = Bundle(cluster=w153, "STATUS"=w154) -> (w152:T4)  [unwired: 2 in]
          n119 = Bundle(cluster=w159, "STATUS"=w161) -> (w160:T4)  [unwired: 2 in]
          n120 = Bundle(cluster=w168, "STATUS"=w167) -> (w166:T4)  [unwired: 2 in]
          n121 = local write "DISP LAB01-2"(w160) -> ()
          n122 = local write "DISP LAB01-1"(w166) -> ()
          n123 = local write "DISP LAB02-1"(w152) -> ()
          n124 = local write "DISP LAB03-1"(w138) -> ()
          n125 = local write "DISP LAB02-2"(w145) -> ()
          n126 = local write "DISP LAB03-2"(w131) -> ()
          n127 = local read "DISP LAB05-2"() -> (w104:T4)
          n128 = local read "DISP LAB05-1"() -> (w111:T4)
          n129 = local read "DISP LAB04-2"() -> (w113:T4)
          n130 = local read "DISP LAB04-1"() -> (w115:T4)
          n131 = Unbundle(w104) -> ("STATUS"=w106:string)  [unwired: 2 out]
          n132 = Unbundle(w111) -> ("STATUS"=w117:string)  [unwired: 2 out]
          n133 = Unbundle(w113) -> ("STATUS"=w122:string)  [unwired: 2 out]
          n134 = Unbundle(w115) -> ("STATUS"=w127:string)  [unwired: 2 out]
          n135 = Equal?(x="", y=w106) -> (x = y?=w108:bool)
          n136 = Equal?(x="", y=w117) -> (x = y?=w119:bool)
          n137 = Equal?(x="", y=w122) -> (x = y?=w124:bool)
          n138 = Equal?(x="", y=w127) -> (x = y?=w129:bool)
          n139 = Select(t="STOP", s=w108, f=w106) -> (s? t:f=w105:string)
          n140 = Select(t="STOP", s=w119, f=w117) -> (s? t:f=w116:string)
          n141 = Select(t="STOP", s=w124, f=w122) -> (s? t:f=w121:string)
          n142 = Select(t="STOP", s=w129, f=w127) -> (s? t:f=w126:string)
          n143 = Bundle(cluster=w104, "STATUS"=w105) -> (w103:T4)  [unwired: 2 in]
          n144 = Bundle(cluster=w111, "STATUS"=w116) -> (w110:T4)  [unwired: 2 in]
          n145 = Bundle(cluster=w113, "STATUS"=w121) -> (w112:T4)  [unwired: 2 in]
          n146 = Bundle(cluster=w115, "STATUS"=w126) -> (w114:T4)  [unwired: 2 in]
          n147 = local write "DISP LAB05-2"(w103) -> ()
          n148 = local write "DISP LAB05-1"(w110) -> ()
          n149 = local write "DISP LAB04-1"(w114) -> ()
          n150 = local write "DISP LAB04-2"(w112) -> ()
        }
        frame #6 {
          # "initialise analog input express vi's"
          n151 = for {
            N: 2.0 -> [_]
            n152 = call "sub vi - analog 1st setup v1.vi"() -> ("error out"=w175:errorcluster)  [unwired: 11 in, 4 out]
            n153 = Unbundle(w175) -> ("status"=w174:bool)  [unwired: 2 out]
            n154 = local write "simulate"(w174) -> ()
          }
        }
        frame #7 {
          # "get initial temperature values"
          n155 = stacked-sequence {
            frame #0 {
              w214 = TRUE
              n156 = local read "simulate"() -> (w176:bool)
              n157 = call "sub vi - GET ALL TEMP v5.vi"("LA01-EN"=w214, "simulate"=w176, "LA02-EN"=w214, "LA03-EN"=w214, "LA04-EN"=w214, "LA05-EN"=w214, "Gen Cal Value"=1) -> ("LA01 TEMP"=w212:T22, "LA02 TEMP"=w205:T22, "LA03 TEMP"=w198:T22, "LA04 TEMP"=w191:T22, "LA05 TEMP"=w184:T22)  [unwired: 3 in, 1 out]
              n158 = local write "LAB05 TEMP"(w184) -> ()
              n159 = local write "LAB04 TEMP"(w191) -> ()
              n160 = local write "LAB01 TEMP"(w212) -> ()
              n161 = local write "LAB02 TEMP"(w205) -> ()
              n162 = local write "LAB03 TEMP"(w198) -> ()
              n163 = Unbundle(w198) -> ("T1"=w195:dbl, "T2"=w194:dbl, "T3"=w193:dbl, "T4"=w192:dbl)  [unwired: 2 out]
              n164 = Unbundle(w212) -> ("T1"=w210:dbl, "T2"=w209:dbl, "T3"=w208:dbl, "T4"=w207:dbl)  [unwired: 2 out]
              n165 = Unbundle(w205) -> ("T1"=w202:dbl, "T2"=w201:dbl, "T3"=w200:dbl, "T4"=w199:dbl)  [unwired: 2 out]
              n166 = Unbundle(w191) -> ("T1"=w189:dbl, "T2"=w188:dbl, "T3"=w187:dbl, "T4"=w186:dbl)  [unwired: 2 out]
              n167 = Unbundle(w184) -> ("T1"=w182:dbl, "T2"=w181:dbl, "T3"=w180:dbl, "T4"=w179:dbl)  [unwired: 2 out]
              n168 = local read "TEMP LA05"() -> (w183:T8)
              n169 = local read "TEMP LA04"() -> (w190:T8)
              n170 = local write "Temp Loops"(0) -> ()
              n171 = local read "TEMP LA02"() -> (w204:T8)
              n172 = local read "TEMP LA03"() -> (w197:T8)
              n173 = local read "TEMP LA01"() -> (w211:T8)
              n174 = Bundle(cluster=w197, "TL-1"=w195, "TN-1"=w194, "TL-2"=w193, "TN-2"=w192) -> (w196:T8)  [unwired: 4 in]
              n175 = Bundle(cluster=w211, "TL-1"=w210, "TN-1"=w209, "TL-2"=w208, "TN-2"=w207) -> (w206:T8)  [unwired: 4 in]
              n176 = Bundle(cluster=w204, "TL-1"=w202, "TN-1"=w201, "TL-2"=w200, "TN-2"=w199) -> (w203:T8)  [unwired: 4 in]
              n177 = Bundle(cluster=w190, "TL-1"=w189, "TN-1"=w188, "TL-2"=w187, "TN-2"=w186) -> (w185:T8)  [unwired: 4 in]
              n178 = Bundle(cluster=w183, "TL-1"=w182, "TN-1"=w181, "TL-2"=w180, "TN-2"=w179) -> (w178:T8)  [unwired: 4 in]
              n179 = local write "TEMP LA03"(w196) -> ()
              n180 = local write "TEMP LA01"(w206) -> ()
              n181 = local write "TEMP LA02"(w203) -> ()
              n182 = local write "TEMP LA05"(w178) -> ()
              n183 = local write "TEMP LA04"(w185) -> ()
            }
            frame #1 {
              w215 = 0
              n184 = local read "LAB01 TEMP"() -> (w221:T11)
              n185 = Unbundle By Name(w221) -> ("T1 Live"=w220:dbl, "T1 Neut"=w219:dbl, "T2 Live"=w218:dbl, "T2 Neut"=w217:dbl)  [unwired: 2 out]
              n186 = local read "TEMP LA01"() -> (w222:T8)
              n187 = Bundle By Name(cluster=w222, "TL-1"=w220, "TN-1"=w219, "TL-2"=w218, "TN-2"=w217, "TL -1COUNT"=w215, "TN-1 COUNT"=w215, "TL-2 COUNT"=w215, "TN-2 COUNT"=w215) -> (w216:T8)
              n188 = local write "TEMP LA01"(w216) -> ()
            }
            frame #2 {
              w223 = 0
              n189 = local read "LAB02 TEMP"() -> (w229:T11)
              n190 = Unbundle By Name(w229) -> ("T1 Live"=w228:dbl, "T1 Neut"=w227:dbl, "T2 Live"=w226:dbl, "T2 Neut"=w225:dbl)  [unwired: 2 out]
              n191 = local read "TEMP LA02"() -> (w230:T8)
              n192 = Bundle By Name(cluster=w230, "TL-1"=w228, "TN-1"=w227, "TL-2"=w226, "TN-2"=w225, "TL -1COUNT"=w223, "TN-1 COUNT"=w223, "TL-2 COUNT"=w223, "TN-2 COUNT"=w223) -> (w224:T8)
              n193 = local write "TEMP LA02"(w224) -> ()
            }
            frame #3 {
              w231 = 0
              n194 = local read "LAB03 TEMP"() -> (w237:T11)
              n195 = Unbundle By Name(w237) -> ("T1 Live"=w236:dbl, "T1 Neut"=w235:dbl, "T2 Live"=w234:dbl, "T2 Neut"=w233:dbl)  [unwired: 2 out]
              n196 = local read "TEMP LA03"() -> (w238:T8)
              n197 = Bundle By Name(cluster=w238, "TL-1"=w236, "TN-1"=w235, "TL-2"=w234, "TN-2"=w233, "TL -1COUNT"=w231, "TN-1 COUNT"=w231, "TL-2 COUNT"=w231, "TN-2 COUNT"=w231) -> (w232:T8)
              n198 = local write "TEMP LA03"(w232) -> ()
            }
            frame #4 {
              w239 = 0
              n199 = local read "LAB04 TEMP"() -> (w245:T11)
              n200 = Unbundle By Name(w245) -> ("T1 Live"=w244:dbl, "T1 Neut"=w243:dbl, "T2 Live"=w242:dbl, "T2 Neut"=w241:dbl)  [unwired: 2 out]
              n201 = local read "TEMP LA04"() -> (w246:T8)
              n202 = Bundle By Name(cluster=w246, "TL-1"=w244, "TN-1"=w243, "TL-2"=w242, "TN-2"=w241, "TL -1COUNT"=w239, "TN-1 COUNT"=w239, "TL-2 COUNT"=w239, "TN-2 COUNT"=w239) -> (w240:T8)
              n203 = local write "TEMP LA04"(w240) -> ()
            }
            frame #5 {
              w247 = 0
              n204 = local read "LAB05 TEMP"() -> (w253:T11)
              n205 = Unbundle By Name(w253) -> ("T1 Live"=w252:dbl, "T1 Neut"=w251:dbl, "T2 Live"=w250:dbl, "T2 Neut"=w249:dbl)  [unwired: 2 out]
              n206 = local read "TEMP LA05"() -> (w254:T8)
              n207 = Bundle By Name(cluster=w254, "TL-1"=w252, "TN-1"=w251, "TL-2"=w250, "TN-2"=w249, "TL -1COUNT"=w247, "TN-1 COUNT"=w247, "TL-2 COUNT"=w247, "TN-2 COUNT"=w247) -> (w248:T8)
              n208 = local write "TEMP LA05"(w248) -> ()
            }
          }
        }
        frame #8 {
          # "enable front panel, all settings done"
